vi "Enable-Disable Dynamic Shunt Cal.vi"(8 "error in":errorcluster, 10 "Dynamic shunt?":bool, 11 "Node Ptr in":T1 format="%.0x") -> (0 "error out":errorcluster, 3 "Node Ptr out":T1 format="%.0x")   [LabVIEW 2011, in "Modules.lvlib" / "9235.lvclass"]
uses:
  9235.lvclass
  <vilib>/NI Veristand/Custom Device API/Custom Device Item Ref.ctl
  9235.lvclass/9235.ctl
  <vilib>/NI Veristand/Custom Device API/Custom Device Channel.ctl
  <vilib>/NI Veristand/Custom Device API/Custom Device Channel Type.ctl
  RSI Module/Channel GUIDs.vi
  <vilib>/NI Veristand/Custom Device Tools/Custom Device Utility Library/NI VeriStand - Search for Item by GUID.vi
  <vilib>/NI Veristand/Custom Device Tools/Custom Device Utility Library/Custom Device Utility Library.lvlib
  RSI Module/RSI Module.lvclass
  <vilib>/NI Veristand/Custom Device API/Custom Device API.lvlib
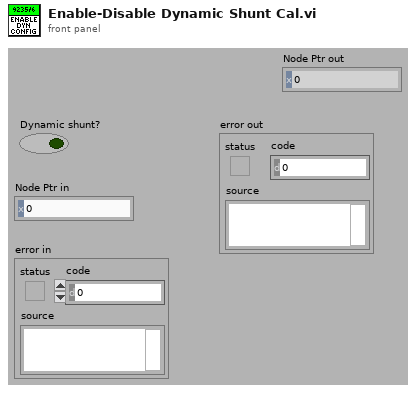
[diagram p1: front panel]
types:
  T1 = typedef "Custom Device API.lvlib/Custom Device Item Ref.ctl" = u64
  T2 = typedef "Custom Device API.lvlib/Custom Device Channel.ctl" = cluster{"Type":T3, "Units":string, "Default Value":dbl, "Faultable":bool, "Scalable":bool}
  T3 = typedef "Custom Device API.lvlib/Custom Device Channel Type.ctl" = enum16{"Input", "Output"}
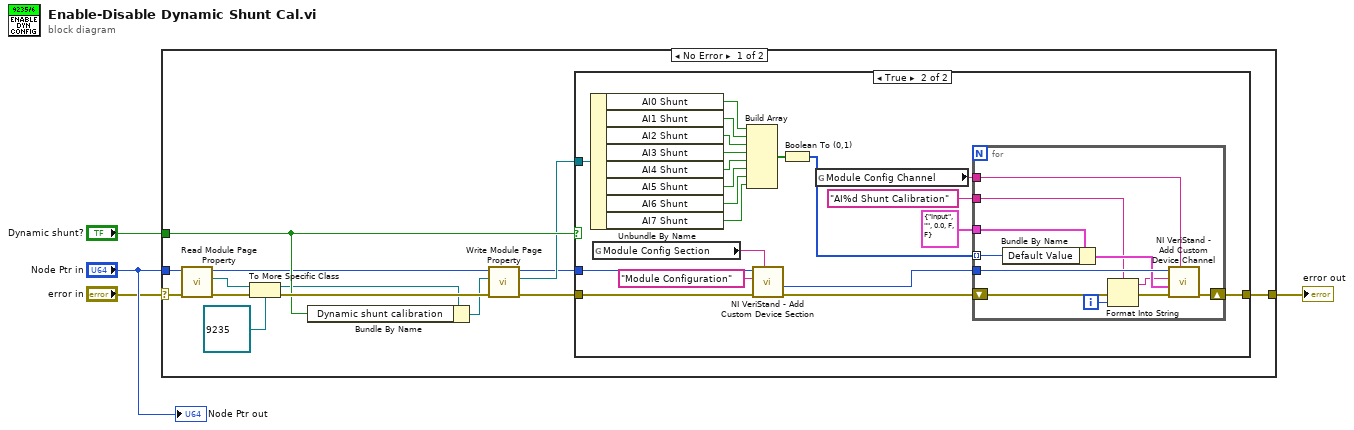
[diagram p0: block diagram]
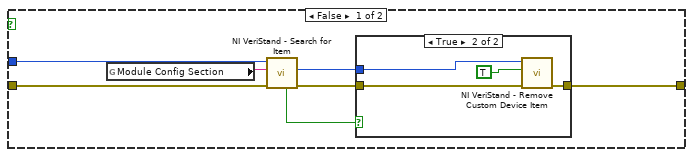
[diagram p2: hidden frame]
diagram:
  n1 = case shown="No Error" "error in" {
    selector: "error in" -> [w16 w63]
    tunnel: [w5 w63] -> w4
    tunnel: "Node Ptr in" -> [w18 _]
    tunnel: "Dynamic shunt?" -> [w12 _]
    frame No Error {
      n2 = call "Read Module Page Property.vi"("error in (no error)"=w16, "Node Ptr In"=w18) -> ("error out"=w15:errorcluster, "RSI Module"=w14:refnum<class "RSI Module.lvclass">, "Node Ptr Out"=w9:T1)  [unwired: 7 in]
      n3 = To More Specific Class(target class=refnum<class "9235.lvclass"> refnum ("9205 in"), reference=w14, error in=w15) -> (specific class reference=w11:refnum<class "9235.lvclass">, error out=w13:errorcluster)
      n4 = Bundle By Name(cluster=w11, "Dynamic shunt calibration"=w12) -> (w10:refnum<class "9235.lvclass">)
      n5 = call "Write Module Page Property.vi"("error in (no error)"=w13, "RSI Module"=w10, "Node Ptr In"=w9) -> ("error out"=w6:errorcluster, "RSI Module out"=w8:refnum<class "9235.lvclass">, "Node Ptr Out"=w7:T1)  [unwired: 6 in]
      n6 = case shown="True" w12 {
        tunnel: w7 -> [w25 w51]
        tunnel: w6 -> [w24 w50]
        tunnel: [w19 w37] -> w5
        tunnel: w8 -> [_ w36]
        frame False {
          n7 = global read "Channel GUIDs.vi" "Module Config Section"() -> (w23:string)
          n8 = call-poly <vilib>:"NI VeriStand - Search for Item.vi"("error in"=w24, "Item GUID"=w23, "Section Ref in"=w25) -> ("error out"=w21:errorcluster, "Item Ref"=w20:T1, "Found"=w22:bool)  [unwired: 5 in, 1 out]
          n9 = case shown="True" w22 {
            tunnel: w21 -> [w26 w30]
            tunnel: w20 -> [_ w29]
            tunnel: [w26 w27] -> w19
            frame False {
            }
            frame True {
              n10 = call <vilib>:"NI VeriStand - Remove Custom Device Item.vi"("error in (no error)"=w30, "Force Delete (F)"=TRUE, "Item Ref in"=w29) -> ("error out"=w27:errorcluster)  [unwired: 7 in, 1 out]
            }
          }
        }
        frame True {
          n11 = Unbundle By Name(w36) -> ("AI0 Shunt"=w45:bool, "AI1 Shunt"=w44:bool, "AI2 Shunt"=w43:bool, "AI3 Shunt"=w42:bool, "AI4 Shunt"=w34:bool, "AI5 Shunt"=w33:bool, "AI6 Shunt"=w32:bool, "AI7 Shunt"=w31:bool)
          n12 = global read "Channel GUIDs.vi" "Module Config Section"() -> (w49:string)
          n13 = Build Array(w45, w44, w43, w42, w34, w33, w32, w31) -> (w40:bool[])
          n14 = call <vilib>:"NI VeriStand - Add Custom Device Section.vi"("GUID (Default Section)"=w49, "error in (no error)"=w50, "Section Name"="Module Configuration", "Parent Ref in"=w51) -> ("error out"=w47:errorcluster, "Section Ptr"=w35:T1)  [unwired: 4 in, 2 out]
          n15 = Boolean To (0,1)(Boolean=w40) -> (0, 1=w39:i16[])
          n16 = global read "Channel GUIDs.vi" "Module Config Channel"() -> (w46:string)
          n17 = for {
            tunnel: w35 -> [w62]
            shift-right: [w61] -> w37
            shift-left: w47 -> [w54]
            tunnel: w46 -> [w60]
            tunnel: T2 {"Type"=enum."Input", "Units"="", "Default Value"=0.0, "Faultable"=FALSE, "Scalable"=FALSE} ("Channel") -> [w59]
            tunnel: w39 -> [w58] mode=indexing
            tunnel: "AI%d Shunt Calibration" ("Channel Name") -> [w56]
            i -> [w55]
            n18 = Bundle By Name(cluster=w59, "Default Value"=w58) -> (w57:T2)
            n19 = Format Into String(format string=w56, error in=w54, w55) -> (resulting string=w52:string, error out=w53:errorcluster)  [unwired: 1 in]
            n20 = call <vilib>:"NI VeriStand - Add Custom Device Channel.vi"("GUID (Default Channel)"=w60, "error in (no error)"=w53, "Channel"=w57, "Channel Name"=w52, "Parent Ref in"=w62) -> ("error out"=w61:errorcluster)  [unwired: 3 in, 3 out]
          }
        }
      }
    }
    frame Error {
    }
  }
  "error out" <- w4
  "Node Ptr out" <- "Node Ptr in"
